vi "fisiere_v7.vi"() -> ()   [LabVIEW 2009]
panel:
  out "txt_wr":string
  out "Nr_stud":u8=4 max=10 step=1
  in  "Calea si numele fisierului":path=path "E:/Projects/Lab_view/Proiecte_concurs/Project 4/Winners.txt"
  out "Studenti":string[][](array[string])
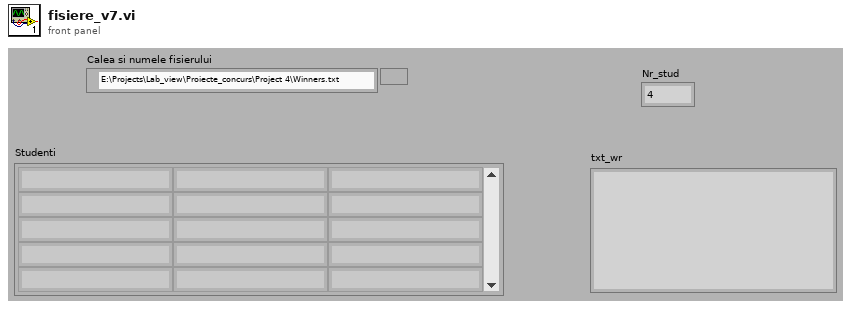
[diagram p1: front panel]
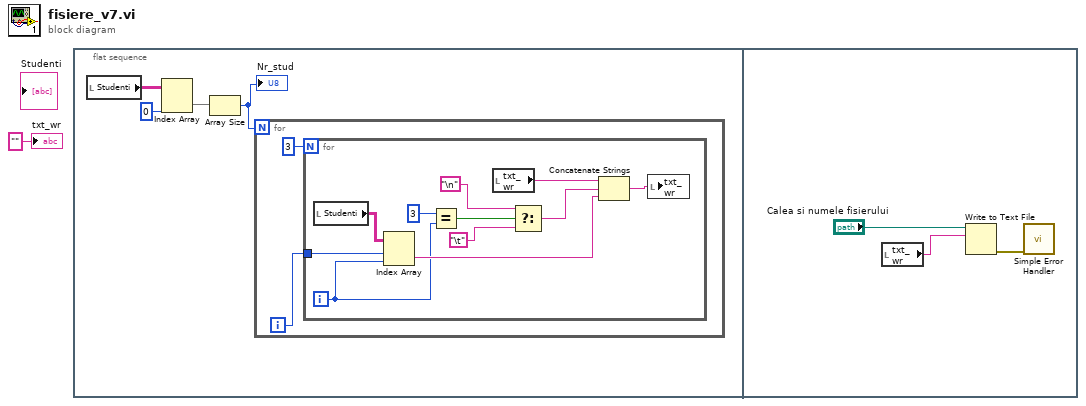
[diagram p0: block diagram]
diagram:
  n1 = flat-sequence {
    frame #0 {
      n2 = local read "Studenti"() -> (w5:string[][])
      n3 = Index Array(array=w5, index (col)=0 ("disabled index (col)")) -> (element=w4:string[])  [unwired: 1 in]
      n4 = Array Size(array=w4) -> (size(s)=w3:i32)
      "Nr_stud" <- w3
      n5 = for {
        N: w3 -> [_]
        i -> [w7]
        n6 = for {
          N: 3 -> [_]
          tunnel: w7 -> [w18]
          i -> [w10]
          n7 = local read "Studenti"() -> (w15:string[][])
          n8 = Index Array(array=w15, index (row)=w18, index (col)=w10) -> (element=w14:string)
          n9 = Equal?(x=3, y=w10) -> (x = y?=w8:bool)
          n10 = local read "txt_wr"() -> (w16:string)
          n11 = Select(t="\n", s=w8, f="\t") -> (s? t:f=w13:string)
          n12 = Concatenate Strings(w16, w13, w14) -> (w17:string)
          n13 = local write "txt_wr"(w17) -> ()
        }
      }
    }
    frame #1 {
      n14 = local read "txt_wr"() -> (w19:string)
      n15 = Write to Text File(file (use dialog)="Calea si numele fisierului", text=w19) -> (error out=w20:errorcluster)  [unwired: 2 in, 2 out]
      n16 = call <vilib>:"Simple Error Handler.vi"("error in (no error)"=w20) -> ()  [unwired: 4 in, 5 out]
    }
  }
  "txt_wr" <- "" ("txt_wr")
